vi "XML Parse Array.vi"(7 "error in (no error)":errorcluster, 8 "Name String":string, 9 "Type String":string, 10 "Path":path) -> (0 "error out":errorcluster, 2 "Array":string[](array[string]))   [LabVIEW 2015]
uses:
  <vilib>/xml/Load XML File.vi
  <vilib>/xml/NI_XML.lvlib
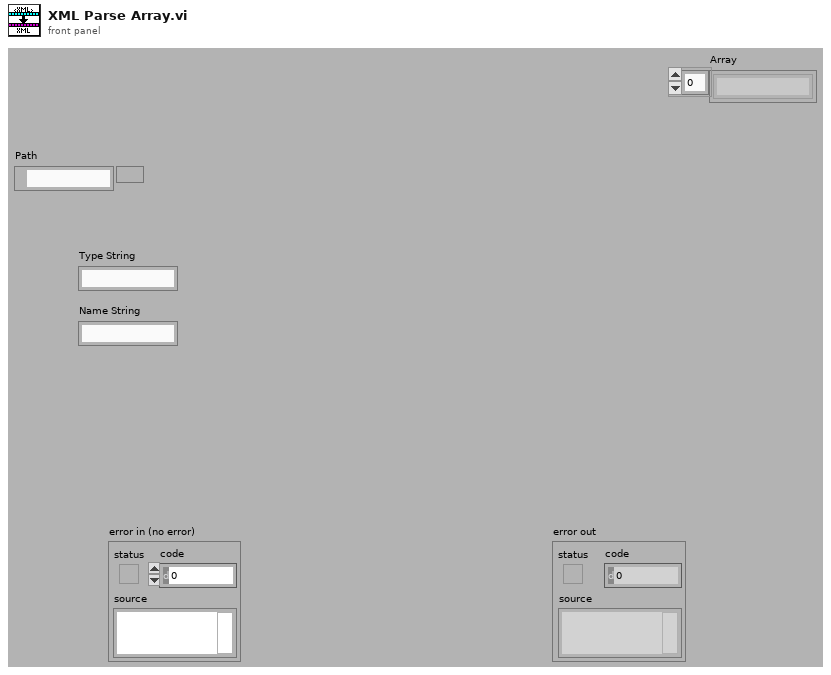
[diagram p1: front panel]
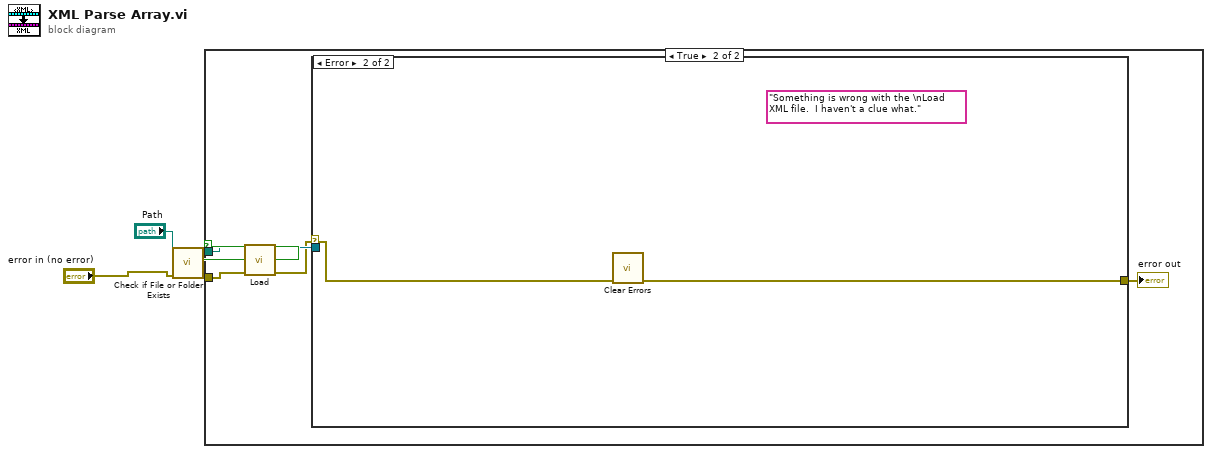
[diagram p0: block diagram]
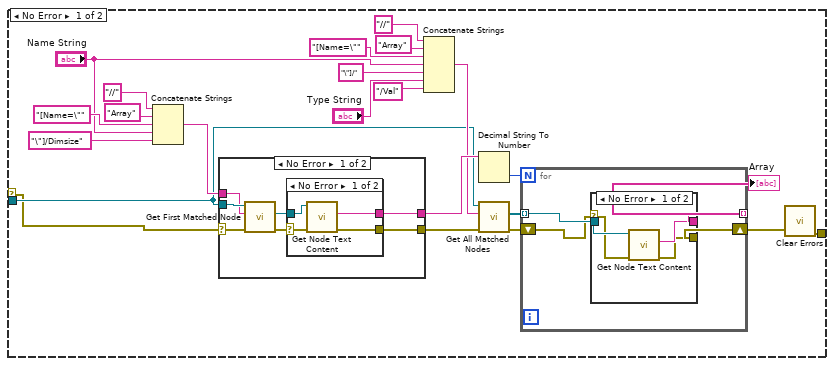
[diagram p3: hidden frame]
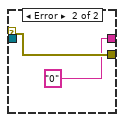
[diagram p4: hidden frame]
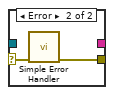
[diagram p5: hidden frame]
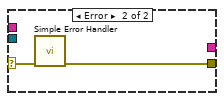
[diagram p6: hidden frame]
diagram:
  n1 = call <vilib>:"Check if File or Folder Exists.vi"("error in (no error)"="error in (no error)", "path"="Path") -> ("error out"=w3:errorcluster, "file or folder exists?"=w1:bool, "dup path"=w4:path)  [unwired: 7 in]
  n2 = case shown="True" w1 {
    tunnel: w3 -> [_ w10]
    tunnel: w4 -> [_ w9]
    frame False {
    }
    frame True {
      n3 = call-poly <vilib>:"Load.vi"("path to XML document"=w9, "error in (no error)"=w10) -> ("DOM document out"=w8:refnum<k20>, "error out"=w6:errorcluster)  [unwired: 11 in, 1 out]
      n4 = case shown="Error" w6 {
        selector: w6 -> [w11 w60]
        tunnel: w8 -> [w18 _]
        tunnel: [w12 w59] -> w7
        frame No Error {
          n5 = Concatenate Strings("//", "Array", "[Name=\"", "Name String", "\"]/Dimsize") -> (w30:string)
          n6 = case shown="No Error" w11 {
            selector: w11 -> [w48 w58]
            tunnel: w18 -> [w50 _]
            tunnel: w30 -> [w49 _]
            tunnel: [w46 _] -> w28
            tunnel: [w45 w57] -> w17
            frame No Error {
              n7 = call <vilib>:"Get First Matched Node.vi"("error in (no error)"=w48, "XPath expression"=w49, "node in"=w50) -> ("error out"=w47:errorcluster, "node result"=w44:refnum<k20>)  [unwired: 6 in, 1 out]
              n8 = case shown="No Error" w47 {
                selector: w47 -> [w53 w56]
                tunnel: w44 -> [w54 _]
                tunnel: [w52 _] -> w46
                tunnel: [w51 w55] -> w45
                frame No Error {
                  n9 = call <vilib>:"Get Node Text Content.vi"("error in (no error)"=w53, "node in"=w54) -> ("error out"=w51:errorcluster, "node text"=w52:string)  [unwired: 7 in, 1 out]
                }
                frame Error {
                  n10 = call <vilib>:"Simple Error Handler.vi"("error in (no error)"=w56) -> ("error out"=w55:errorcluster)  [unwired: 4 in, 4 out]
                }
              }
            }
            frame Error {
              n11 = call <vilib>:"Simple Error Handler.vi"("error in (no error)"=w58) -> ("error out"=w57:errorcluster)  [unwired: 4 in, 4 out]
            }
          }
          n12 = Concatenate Strings("//", "Array", "[Name=\"", "Name String", "\"]/", "Type String", "/Val") -> (w19:string)
          n13 = Decimal String To Number(string=w28) -> (number=w27:i32)  [unwired: 2 in, 1 out]
          n14 = call <vilib>:"Get All Matched Nodes.vi"("error in (no error)"=w17, "XPath expression"=w19, "node in"=w18) -> ("error out"=w14:errorcluster, "node result array"=w16:refnum<k20>[])  [unwired: 6 in, 1 out]
          n15 = for {
            N: w27 -> [_]
            tunnel: w16 -> [w37] mode=indexing
            tunnel: [w36] -> w15 mode=indexing
            shift-right: [w35] -> w13
            shift-left: w14 -> [w34]
            n16 = case shown="No Error" w34 {
              selector: w34 -> [w38 w43]
              tunnel: w37 -> [w41 _]
              tunnel: [w40 "0"] -> w36
              tunnel: [w39 w43] -> w35
              frame No Error {
                n17 = call <vilib>:"Get Node Text Content.vi"("error in (no error)"=w38, "node in"=w41) -> ("error out"=w39:errorcluster, "node text"=w40:string)  [unwired: 7 in, 1 out]
              }
              frame Error {
              }
            }
          }
          "Array" <- w15
          n18 = call <vilib>:"Clear Errors.vi"("error in (no error)"=w13) -> ("error out"=w12:errorcluster)  [unwired: 5 in, 1 out]
        }
        frame Error {
          (unwired) "Something is wrong with the \nLoad XML file.  I haven't a clue what."
          n19 = call <vilib>:"Clear Errors.vi"("error in (no error)"=w60) -> ("error out"=w59:errorcluster)  [unwired: 5 in, 1 out]
        }
      }
      "error out" <- w7
    }
  }
